vi "final_control_mk4_022525.vi"() -> ()   [LabVIEW 2023]
doc: "Simplified example program for initializing the COM port, determining the data frame of up to 26 Alicats, acquiring the data of the same number of Alicats, displaying the data of the one with the selected unit ID, and writing a setpoint to the same selected unit ID.\n\nThis is a slightly more feature rich version of the Alicat Simplified Driver Example, and contains an example of a method for interfacing with up to 26 Alicats on a single COM port by means of for loops with shift registers to handle sequential commands to each included Alicat. This also contains a method to write a setpoint to the same selected unit.\n\nIf coding for multiple Alicats on a single COM port without the use of for loops with shift registers, ensure that each Alicat command is executed sequentially. Alicat's RS-232/485 does not work if multiple devices are responding simultaneously."
uses:
  <vilib>/Platform/TimedLoop/XDataNode/timing_clust.ctl
  <vilib>/Platform/TimedLoop/XDataNode/nitl_modes.ctl
  <vilib>/Platform/TimedLoop/XDataNode/wakeup.ctl
  <vilib>/DAQmx/write.llb/DAQmx Write (Analog 1D DBL NChan 1Samp).vi
  <vilib>/DAQmx/read.llb/DAQmx Read (Analog 1D DBL 1Chan NSamp).vi
  <extravilib>/ChannelInstances/Tag-bool/Read With Abort.vi
  <extravilib>/ChannelInstances/Tag-bool/Write With Abort.vi
  <vilib>/Utility/file.llb/Write Delimited Spreadsheet (string).vi
  <extravilib>/ChannelInstances/Tag-bool/Instantiate.vi
  <vilib>/Utility/file.llb/Read Delimited Spreadsheet (DBL).vi
  <extravilib>/ChannelInstances/Tag-bool/EndpointRead.vi
  <vilib>/DAQmx/miscellaneous.llb/DAQmx Fill In Error Info.vi
  <extravilib>/ChannelInstances/Tag-bool/Endpoint.vi
  <vilib>/platform/TimedLoop/XDataNode/XDataNode.xnode
  <vilib>/Platform/TimedLoop/XDataNode/XDNodeRunTimeDep.lvlib
  <extravilib>/ChannelInstances/Tag-bool.lvlib
panel:
  in  "Tab Control":enum32{"Page 1", "Page 2"}(tab)
  in  "COM Port Settings":T1={"Baud Rate"=enum."19200", "VISA Sesssion In"="COM1"}
  out "Range Exceeded":bool
  out "Error Present":bool
  out "Error Text":string
  out "Elapsed Time [ms]\n(all units)":dbl caption="Elapsed Time (s)"
  in  "Minimum time between \nreadings [ms] (all units)":u32
  in  "Device ID's \nto Include:":T2={"A"=TRUE, "B"=FALSE, "C"=FALSE, "D"=FALSE, "E"=FALSE, "F"=FALSE, "G"=FALSE, "H"=FALSE, "I"=FALSE, "J"=FALSE, "K"=FALSE, "L"=FALSE, "M"=FALSE, "N"=FALSE, "O"=FALSE, "P"=FALSE, "Q"=FALSE, "R"=FALSE, "S"=FALSE, "T"=FALSE, "U"=FALSE, "V"=FALSE, "W"=FALSE, "X"=FALSE, "Y"=FALSE, "Z"=FALSE}
  out "Active Device":u16(ring) items=["A", "B", "C", "D", "E", "F"]
  out "Meas. Data (for active device)":T3
  in  "Write File":path=path "C:/Users/gtmiller/Downloads/Alicat LabVIEW 2014_2v1/Test.csv"
  in  "Hold Time [min]":dbl=17.0 min=17.0
  out "Global Start Time":i64
  out "N":i32
  out "Iteration Duration":i64
  in  "Read File":path
  in  "End Program":bool
  out "len_SP":i32
  out "Setpoints":dbl[][](array[numeric])=[[4.2, 3.3], [69.0, 4.2]]
  out "Z":dbl[](array[numeric])
  out "ASP":dbl
  out "BSP":dbl
  out "CSP":dbl
  out "DSP":dbl
  out "ESP":dbl
  out "FSP":dbl
  out "N_i_read":dbl
  out "N_read":i32
  out "read count":dbl=2.0
  out "Actual Start [i]":i64
  out "T_SCh":string[](array[string])
  out "Iter_Start_Time":string
  out "Iter_#":string
  out "V_D":string
  out "V_H":string
  # "Totalizer Timer"
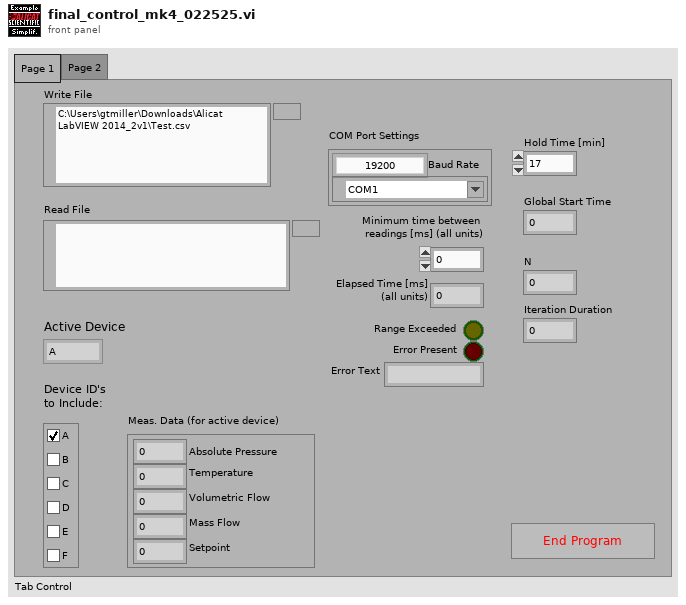
[diagram p1: front panel]
types:
  T1 = cluster{"Baud Rate":enum8{"2400", "9600", "19200", "38400", "57600", "115200", "Unknown"}, "VISA Sesssion In":refnum<visa-resource-name>}
  T2 = cluster{"A":bool, "B":bool, "C":bool, "D":bool, "E":bool, "F":bool, "G":bool, "H":bool, "I":bool, "J":bool, "K":bool, "L":bool, "M":bool, "N":bool, "O":bool, "P":bool, "Q":bool, "R":bool, "S":bool, "T":bool, "U":bool, "V":bool, "W":bool, "X":bool, "Y":bool, "Z":bool}
  T3 = cluster{"Absolute Pressure":dbl, "Gauge/Diff. Pressure":dbl, "Barometric Pressure":dbl, "Temperature":dbl, "Volumetric Flow":dbl, "Mass Flow":dbl, "Setpoint":dbl, "Valve Drive":dbl, "Totalizer":dbl, "[hr]":dbl, "[min]":dbl, "[sec]":dbl, "Totalizer Average Flow":dbl, "Totalizer Peak Flow":dbl, "Gas selected":string}
  T4 = cluster{"Unit ID":string, "Baud Rate":enum8{"2400", "9600", "19200", "38400", "57600", "115200", "Unknown"}, "VISA Sesssion In":refnum<visa-resource-name>}
  T5 = typedef "XDNodeRunTimeDep.lvlib/timing_clust.ctl" = cluster{"Expected End [f-1]":u64, "Actual End [f-1]":u64, "Finished Late? [f-1]":bool, "Expected End [i-1]":u64, "Actual End [i-1]":u64, "Finished Late? [i-1]":bool, "Expected Start [i]":u64, "Actual Start [i]":u64, "Expected Start [f]":u64, "Actual Start [f]":u64, "Source Name":string, "Structure Name":string, "Period":i64, "Deadline":i64, "Offset":i64, "Start":i64, "Priority":i32, "Timeout":i32, "Mode":T6, "Wakeup Reason":T7, "Error":errorcluster, "Source Type":string, "Secondary Source Type":string, "Global End Time":u64, "Global Start Time":u64, "Frame Duration":u64, "Iteration Duration":u64, "Assigned CPU":i32, "I/O Scan Engine Mode":u32}
  T6 = typedef "XDNodeRunTimeDep.lvlib/nitl_modes.ctl" = enum32{"No Change", "Process missed periods, maintain original phase", "Discard missed periods, maintain original phase", "Process missed periods, ignore original phase", "Discard missed periods, ignore original phase"}
  T7 = typedef "XDNodeRunTimeDep.lvlib/wakeup.ctl" = enum32{"Normal", "Aborted", "Asynchronous wakeup", "Timing source error", "Timed loop error", "Timeout"}
  T8 = enum8{"2400", "9600", "19200", "38400", "57600", "115200", "Unknown"}
  T9 = cluster{"Absolute Pressure":bool, "Gauge/Diff. Pressure":bool, "Barometric Pressure":bool, "Temperature":bool, "Volumetric":bool, "Mass":bool, "Setpoint":bool, "Valve Drive":bool, "Totalizer":bool, "Totalizer Timer":bool, "Totalizer Average Flow":bool, "Totalizer Peak Flow":bool, "Gas Selected":bool, "Tot. Timer Format":u16}
  T10 = cluster{"Controller Full Scale":dbl, "Controller Select":u16, "Control Range":enum16{"Normal", "Inverted", "Bidirectional", "Unknown"}}
  T11 = typedef "Tag-bool.lvlib/))Channel.ctl" = refnum<queue>
  T12 = cluster{"Controller Full Scale":dbl, "Controller Select":u16, "Control Range":enum16{"Normal", "Inverted", "Bidirectional", "Unknown"}}[]
diagram:
  n1 = for {
    N: 1 -> [_]
    # "Initialize Data Hold Array"
    # "All successive for loops to perform\nthe same task to all devices on the\nCOM port can make use of the for\nloop's auto-indexing feature"
    # "Set to run 26 times\n(once per letter)"
    # "Acquisition of data from multiple Alicats on a single serial line requires that the commands and returns are performed sequentially.\nThis is performed using for loops to gather and index the data in a sequential manner, but it can also be done with duplicated VI's called\nsequentially (but this becomes much more tedious if talking to more than 2 devices on a given COM port)."
    # "Numbers paired with Unit ID's included begin at\n0 for ease of use later on with for loop indexes"
    # "Get array of unit ID's and populate the Unit ID control before next step"
    # "Needs to be set before running software ->"
    # "Close the VISA session"
    # "Initialize the Com port\n(cluster bundle/unbundle\nused to provide Sub-VI \nwith the expected input)"
    n2 = Unbundle("COM Port Settings") -> ("Baud Rate"=w34:T8, "VISA Sesssion In"=w33:refnum<visa-resource-name>)
    n3 = Bundle(cluster=T4 {"Unit ID"="A", "Baud Rate"=enum."19200", "VISA Sesssion In"="COM1"} ("Communication Settings"), "Baud Rate"=w34, "VISA Sesssion In"=w33) -> (w32:T4)  [unwired: 1 in]
    n4 = Cluster To Array(cluster="Device ID's \nto Include:") -> (array=w28:bool[])
    n5 = call "COM Port Initialization.vi"("error in (no error)"=errorcluster {"status"=FALSE, "code"=0, "source"=""}, "Communication Settings"=w32) -> ("error out"=w25:errorcluster, "VISA Session Out"=w24:refnum<visa-resource-name>)  [unwired: 8 in]
    n6 = for {
      N: 6 -> [_]
      tunnel: "ABCDEF" -> [w516]
      tunnel: w28 -> [w509] mode=indexing
      shift-right: [w508] -> _
      shift-left: u16 0 ("length (rest)") -> [w514]
      shift-right: [w513] -> w22
      shift-left: cluster{string, u16}[] [] -> [w512]
      tunnel: w25 -> [w507]
      tunnel: w24 -> [w506]
      tunnel: [w507] -> w15
      tunnel: [w506] -> w23
      i -> [w515]
      # "Generate array of Device ID's, with sequential ID's"
      n7 = Equal?(x=w509, y=TRUE) -> (x = y?=w511:bool)
      n8 = case shown="True" w511 {
        tunnel: w516 -> [_ w527]
        tunnel: w515 -> [_ w526]
        tunnel: w514 -> [w517 w519]
        tunnel: [w518 w522] -> w513
        tunnel: w512 -> [w518 w520]
        tunnel: [w517 w523] -> w508
        frame False {
          # "ID was not included"
        }
        frame True {
          # "ID was included"
          n9 = String Subset(string=w527, offset (0)=w526, length (rest)=1 ("length (rest)")) -> (substring=w524:string)
          n10 = Bundle(w524, "length (rest)"=w519) -> (w521:cluster{string, "length (rest)":u16})  [unwired: 1 in]
          n11 = Increment(x=w519) -> (x+1=w523:u16)
          n12 = Build Array (concatenate)(w520, w521) -> (w522:cluster{string, "length (rest)":u16}[])
        }
      }
    }
    n13 = property on="Active Device" class="Ring (strict)"(error in=w15, "StringsAndValues[]"=w22) -> (error out=w14:errorcluster)  [unwired: 1 in, 1 out]
    n14 = for {
      tunnel: w23 -> [w504]
      tunnel: [w501] -> w19
      tunnel: w14 -> [w505]
      tunnel: [w500] -> w18
      tunnel: w22 -> [w502] mode=indexing
      tunnel: [w503] -> w21 mode=indexing
      tunnel: [w493] -> w20 mode=indexing
      tunnel: [w499] -> w17 mode=indexing
      tunnel: [nan ("Setpoint")] -> w16 mode=indexing
      tunnel: [w492] -> w13 mode=indexing
      # "Get measurement formats, unit ID's and the controller info"
      n15 = Unbundle(w502) -> (w493:string)  [unwired: 1 out]
      n16 = call "Read Measurement Format.vi"("Unit ID (A)"=w493, "error in"=w505, "VISA Session In"=w504) -> ("error out"=w496:errorcluster, "Data Frame Format"=w503:T9, "VISA Session Out"=w497:refnum<visa-resource-name>)  [unwired: 6 in]
      n17 = property on="Active Device" class="Ring (strict)" props=["Value"]() -> ()  [unwired: 2 in, 3 out]
      n18 = call "Read Software Version.vi"("Unit ID (A)"=w493, "error in"=w496, "VISA Session In"=w497) -> ("error out"=w495:errorcluster, "Software Version"=w492:u8, "VISA Session Out"=w494:refnum<visa-resource-name>)  [unwired: 6 in]
      n19 = call "Read Controller Info.vi"("Unit ID (A)"=w493, "error in"=w495, "Software Version"=w492, "VISA Session In"=w494) -> ("error out"=w500:errorcluster, "Controller Info out"=w499:T10, "VISA Session Out"=w501:refnum<visa-resource-name>)  [unwired: 4 in, 1 out]
    }
    n20 = Multiply(x="Hold Time [min]", y=60000.0) -> (x*y=w2:dbl)
    n21 = node-c288(w2) -> (w43:T5)  [unwired: 3 in]
    n22 = timed-loop "Write Data" {
      timing: w43 -> [_]
      timing-out: [_] -> w42
      tunnel: [w54] -> w9
      tunnel: "Write File" -> [w53]
      i -> [w66]
      stop <- w194 stop-if-true
      n23 = timed-sequence {
        timing: _ -> [_]
        timing-out: _ -> [_]
        tunnel: [w56] -> w54
        tunnel: w53 -> [w55]
        n24 = timed-flat-sequence {
          tunnel: [w189] -> w56
          tunnel: w55 -> [w190]
          frame #0 {
            w59 = u16 0 items=["A", "B", "C", "D", "E", "F"]
            n25 = node-c288() -> (→"Global Start Time":i64, →"Iteration Duration":i64)  [unwired: 1 in]
            n26 = local read "Setpoints"() -> (w68:dbl[][])
            n27 = Index Array(array=w68, index (row)=w66, index (col)=0 ("index (row)")) -> (element=w64:dbl)
            "ASP" <- w64
            n28 = local read "Z"() -> (w62:dbl[])
            n29 = Replace Array Subset(array=w62, new element #1=w64, index #1=0 ("index"), new element #2=w59, index #2=1 ("index")) -> (w63:dbl[])
            n30 = local write "Z"(w63) -> ()
            n31 = node-c288(i64 2000 ("Start")) -> ()  [unwired: 1 out]
            "N" <- w66
          }
          frame #1 {
            w77 = u16 1 items=["A", "B", "C", "D", "E", "F"]
            n32 = node-c288() -> ()  [unwired: 1 in, 1 out]
            n33 = local read "Setpoints"() -> (w85:dbl[][])
            n34 = local read "N"() -> (w78:i32)
            n35 = Index Array(array=w85, index (row)=w78, index (col)=1 ("index (row)")) -> (element=w82:dbl)
            "BSP" <- w82
            n36 = local read "Z"() -> (w80:dbl[])
            n37 = Replace Array Subset(array=w80, new element #1=w82, index #1=0 ("index"), new element #2=w77, index #2=1 ("index")) -> (w81:dbl[])
            n38 = call-poly <vilib>:"DAQmx Write.vi"("task/channels in"=refnum<k21> "Valve_cont", "data"=dbl[] [5.0, 5.0]) -> ()  [unwired: 11 in, 3 out]
            n39 = local write "Z"(w81) -> ()
            n40 = node-c288(i64 2000 ("Start")) -> ()  [unwired: 1 out]
          }
          frame #2 {
            w111 = u16 2 items=["A", "B", "C", "D", "E", "F"]
            n41 = node-c288() -> ()  [unwired: 1 in, 1 out]
            n42 = local read "Setpoints"() -> (w94:dbl[][])
            n43 = local read "N"() -> (w93:i32)
            n44 = Index Array(array=w94, index (row)=w93, index (col)=2 ("index (row)")) -> (element=w115:dbl)
            "CSP" <- w115
            n45 = Index Array(array=w94, index (row)=w93, index (col)=6 ("disabled index (col)")) -> (element=w92:dbl)
            n46 = Index Array(array=w94, index (row)=w93, index (col)=7 ("disabled index (col)")) -> (element=w91:dbl)
            n47 = local read "Z"() -> (w113:dbl[])
            n48 = Subtract(x=5.0, y=w92) -> (x-y=w108:dbl)
            n49 = Subtract(x=5.0, y=w91) -> (x-y=w103:dbl)
            n50 = Replace Array Subset(array=w113, new element #1=w115, index #1=0 ("index"), new element #2=w111, index #2=1 ("index")) -> (w114:dbl[])
            n51 = Multiply(x=w108, y=0.33) -> (x*y=w106:dbl)
            n52 = Multiply(x=w103, y=0.33) -> (x*y=w101:dbl)
            n53 = local write "Z"(w114) -> ()
            n54 = Subtract(x=5.0, y=w106) -> (x-y=w96:dbl)
            n55 = Subtract(x=5.0, y=w101) -> (x-y=w97:dbl)
            n56 = Build Array(w96, w97) -> (w95:dbl[])
            n57 = call-poly <vilib>:"DAQmx Write.vi"("task/channels in"=refnum<k21> "Valve_cont", "data"=w95) -> ()  [unwired: 11 in, 3 out]
            n58 = node-c288(i64 2000 ("Start")) -> ()  [unwired: 1 out]
          }
          frame #3 {
            w143 = u16 3 items=["A", "B", "C", "D", "E", "F"]
            n59 = node-c288() -> ()  [unwired: 1 in, 1 out]
            n60 = local read "Setpoints"() -> (w126:dbl[][])
            n61 = local read "N"() -> (w125:i32)
            n62 = Index Array(array=w126, index (row)=w125, index (col)=3 ("index (row)")) -> (element=w147:dbl)
            "DSP" <- w147
            n63 = Index Array(array=w126, index (row)=w125, index (col)=6 ("disabled index (col)")) -> (element=w124:dbl)
            n64 = Index Array(array=w126, index (row)=w125, index (col)=7 ("disabled index (col)")) -> (element=w123:dbl)
            n65 = local read "Z"() -> (w145:dbl[])
            n66 = Subtract(x=5.0, y=w124) -> (x-y=w140:dbl)
            n67 = Subtract(x=5.0, y=w123) -> (x-y=w135:dbl)
            n68 = Replace Array Subset(array=w145, new element #1=w147, index #1=0 ("index"), new element #2=w143, index #2=1 ("index")) -> (w146:dbl[])
            n69 = Multiply(x=w140, y=0.67) -> (x*y=w138:dbl)
            n70 = Multiply(x=w135, y=0.67) -> (x*y=w133:dbl)
            n71 = local write "Z"(w146) -> ()
            n72 = Subtract(x=5.0, y=w138) -> (x-y=w128:dbl)
            n73 = Subtract(x=5.0, y=w133) -> (x-y=w129:dbl)
            n74 = Build Array(w128, w129) -> (w127:dbl[])
            n75 = call-poly <vilib>:"DAQmx Write.vi"("task/channels in"=refnum<k21> "Valve_cont", "data"=w127) -> ()  [unwired: 11 in, 3 out]
            n76 = node-c288(i64 2000 ("Start")) -> ()  [unwired: 1 out]
          }
          frame #4 {
            w164 = u16 4 items=["A", "B", "C", "D", "E", "F"]
            n77 = node-c288() -> ()  [unwired: 1 in, 1 out]
            n78 = local read "Setpoints"() -> (w158:dbl[][])
            n79 = local read "N"() -> (w157:i32)
            n80 = Index Array(array=w158, index (row)=w157, index (col)=4 ("index (row)")) -> (element=w168:dbl)
            "ESP" <- w168
            n81 = Index Array(array=w158, index (row)=w157, index (col)=6 ("disabled index (col)")) -> (element=w160:dbl)
            n82 = Index Array(array=w158, index (row)=w157, index (col)=7 ("disabled index (col)")) -> (element=w159:dbl)
            n83 = local read "Z"() -> (w166:dbl[])
            n84 = Build Array(w160, w159) -> (w156:dbl[])
            n85 = Replace Array Subset(array=w166, new element #1=w168, index #1=0 ("index"), new element #2=w164, index #2=1 ("index")) -> (w167:dbl[])
            n86 = call-poly <vilib>:"DAQmx Write.vi"("task/channels in"=refnum<k21> "Valve_cont", "data"=w156) -> ()  [unwired: 11 in, 3 out]
            n87 = local write "Z"(w167) -> ()
            n88 = node-c288(i64 2000 ("Start")) -> ()  [unwired: 1 out]
          }
          frame #5 {
            w178 = u16 5 items=["A", "B", "C", "D", "E", "F"]
            n89 = node-c288() -> ()  [unwired: 1 in, 1 out]
            n90 = local read "N"() -> (w176:i32)
            n91 = local read "Setpoints"() -> (w181:dbl[][])
            n92 = local read "Z"() -> (w180:dbl[])
            n93 = Index Array(array=w181, index (row)=w176, index (col)=5 ("index (row)")) -> (element=w177:dbl)
            "FSP" <- w177
            n94 = Replace Array Subset(array=w180, new element #1=w177, index #1=0 ("index"), new element #2=w178, index #2=1 ("index")) -> (w179:dbl[])
            n95 = local write "Z"(w179) -> ()
            n96 = node-c288(i64 2000 ("Start")) -> ()  [unwired: 1 out]
          }
          frame #6 {
            n97 = node-c288() -> ()  [unwired: 1 in, 1 out]
            n98 = local read "len_SP"() -> (w193:i32)
            n99 = Subtract(x=w193, y=1) -> (x-y=w196:i32)
            n100 = local read "N"() -> (w192:i32)
            n101 = Equal?(x=w192, y=w196) -> (x = y?=w195:bool)
            n102 = Or(x="End Program", y=w195) -> (x .or. y?=w194:bool)
            n103 = call <extravilib>:"Write.vi"("element"=w194) -> ("channel"=w189:T11)  [unwired: 1 out]
            n104 = while {
              tunnel: w190 -> [w212]
              tunnel: w189 -> [w206]
              i -> [w202]
              stop <- w201 stop-if-true
              w207 = 42.0 ("y")
              # "Read Data"
              n105 = local read "N_i_read"() -> (w199:dbl)
              n106 = node-c288(w199) -> (w214:T5)  [unwired: 3 in]
              n107 = timed-loop {
                timing: w214 -> [_]
                timing-out: [_] -> w213
                tunnel: w212 -> [w216]
                tunnel: w206 -> [w215]
                i -> [w243]
                stop <- w443 stop-if-true
                n108 = timed-sequence {
                  timing: _ -> [_]
                  timing-out: _ -> [_]
                  tunnel: w216 -> [w223]
                  tunnel: w215 -> [w217]
                  n109 = timed-flat-sequence {
                    tunnel: w223 -> [w246]
                    tunnel: [w246] -> w222
                    tunnel: w222 -> [w286]
                    tunnel: [w286] -> w221
                    tunnel: w221 -> [w325]
                    tunnel: [w325] -> w220
                    tunnel: w220 -> [w364]
                    tunnel: [w364] -> w219
                    tunnel: w219 -> [w403]
                    tunnel: [w403] -> w218
                    tunnel: w218 -> [w450]
                    tunnel: w217 -> [w449]
                    frame #0 {
                      w235 = i16 2 ("precision (6)")
                      w242 = u16 5 items=["A", "B", "C", "D", "E", "F"]
                      w250 = u16 0 items=["A", "B", "C", "D", "E", "F"]
                      w251 = i16 6 ("precision (6)")
                      n110 = node-c288() -> (→"Actual Start [i]":i64)  [unwired: 1 in]
                      n111 = local read "Setpoints"() -> (w232:dbl[][])
                      n112 = local read "Setpoints"() -> (w226:dbl[][])
                      n113 = local read "Meas. Data (for active device)"() -> (w258:T3)
                      n114 = call-poly <vilib>:"DAQmx Read.vi"("task/channels in"=refnum<k21> "T_SCh") -> ("data"=w240:dbl[])  [unwired: 12 in, 2 out]
                      n115 = local read "Actual Start [i]"() -> (w236:i64)
                      n116 = local read "N"() -> (w227:i32)
                      n117 = Index Array(array=w232, index (row)=w227, index (col)=6 ("disabled index (col)")) -> (element=w231:dbl)
                      n118 = Index Array(array=w226, index (row)=w227, index (col)=7 ("disabled index (col)")) -> (element=w228:dbl)
                      n119 = local read "ASP"() -> (w244:dbl)
                      n120 = Unbundle(w258) -> ("Absolute Pressure"=w271:dbl, "Temperature"=w267:dbl, "Volumetric Flow"=w257:dbl, "Mass Flow"=w268:dbl, "Setpoint"=w269:dbl)  [unwired: 10 out]
                      n121 = local read "Z"() -> (w254:dbl[])
                      n122 = Number To Fractional String(number=w271, precision (6)=w251) -> (F-format string=w266:string)  [unwired: 2 in]
                      n123 = Number To Fractional String(number=w267, precision (6)=w251) -> (F-format string=w265:string)  [unwired: 2 in]
                      n124 = Number To Fractional String(number=w257, precision (6)=w251) -> (F-format string=w264:string)  [unwired: 2 in]
                      n125 = Number To Fractional String(number=w268, precision (6)=w251) -> (F-format string=w263:string)  [unwired: 2 in]
                      n126 = Number To Fractional String(number=w269, precision (6)=w251) -> (F-format string=w262:string)  [unwired: 2 in]
                      n127 = Number To Fractional String(number=w240, precision (6)=w235) -> (F-format string=w238:string[])  [unwired: 2 in]
                      "T_SCh" <- w238
                      n128 = Number To Fractional String(number=w236, precision (6)=w235) -> (F-format string=w237:string)  [unwired: 2 in]
                      "Iter_Start_Time" <- w237
                      n129 = Number To Fractional String(number=w227, precision (6)=i16 0) -> (F-format string=w234:string)  [unwired: 2 in]
                      "Iter_#" <- w234
                      n130 = Number To Fractional String(number=w231) -> (F-format string=w230:string)  [unwired: 3 in]
                      "V_D" <- w230
                      n131 = Number To Fractional String(number=w228) -> (F-format string=w229:string)  [unwired: 3 in]
                      "V_H" <- w229
                      n132 = Replace Array Subset(array=w254, new element #1=w250, index #1=1 ("index"), new element #2=w244, index #2=0 ("index")) -> (w252:dbl[])
                      n133 = Number To Fractional String(number=w242, precision (6)=w251) -> (F-format string=w270:string)  [unwired: 2 in]
                      n134 = Get Date/Time In Seconds() -> (seconds since 1Jan1904=w256:timestamp)
                      n135 = Get Date/Time String(seconds (now)=w256, want seconds? (F)=TRUE) -> (date string=w255:string, time string=w272:string)  [unwired: 1 in]
                      n136 = local write "Z"(w252) -> ()
                      n137 = Build Array (concatenate)(w255, w272, w270, w266, w265, w264, w263, w262, w238, w237, w234, w230, w229) -> (w259:string[])
                      n138 = node-c288(i64 1000 ("Start")) -> ()  [unwired: 1 out]
                      n139 = call-poly <vilib>:"Write Delimited Spreadsheet.vi"("file path (dialog if empty)"=w246, "format (%s)"="%.6f" ("format (%.3f)"), "1D data"=w259, "append to file? (new file:F)"=TRUE, "delimiter (\\t)"="," ("delimiter (\\t)")) -> ()  [unwired: 9 in, 2 out]
                      "N_read" <- w243
                    }
                    frame #1 {
                      w283 = u16 0 items=["A", "B", "C", "D", "E", "F"]
                      w293 = u16 1 items=["A", "B", "C", "D", "E", "F"]
                      w294 = i16 6 ("precision (6)")
                      n140 = node-c288() -> ()  [unwired: 1 in, 1 out]
                      n141 = local read "Meas. Data (for active device)"() -> (w291:T3)
                      n142 = Unbundle(w291) -> ("Absolute Pressure"=w311:dbl, "Temperature"=w307:dbl, "Volumetric Flow"=w298:dbl, "Mass Flow"=w308:dbl, "Setpoint"=w309:dbl)  [unwired: 10 out]
                      n143 = Number To Fractional String(number=w311, precision (6)=w294) -> (F-format string=w306:string)  [unwired: 2 in]
                      n144 = Number To Fractional String(number=w307, precision (6)=w294) -> (F-format string=w305:string)  [unwired: 2 in]
                      n145 = Number To Fractional String(number=w298, precision (6)=w294) -> (F-format string=w304:string)  [unwired: 2 in]
                      n146 = Number To Fractional String(number=w308, precision (6)=w294) -> (F-format string=w303:string)  [unwired: 2 in]
                      n147 = Number To Fractional String(number=w309, precision (6)=w294) -> (F-format string=w302:string)  [unwired: 2 in]
                      n148 = local read "BSP"() -> (w284:dbl)
                      n149 = local read "T_SCh"() -> (w282:string[])
                      n150 = local read "Iter_Start_Time"() -> (w281:string)
                      n151 = local read "Iter_#"() -> (w280:string)
                      n152 = local read "V_D"() -> (w279:string)
                      n153 = local read "V_H"() -> (w278:string)
                      n154 = local read "Z"() -> (w290:dbl[])
                      n155 = Replace Array Subset(array=w290, new element #1=w293, index #1=1 ("index"), new element #2=w284, index #2=0 ("index")) -> (w289:dbl[])
                      n156 = Number To Fractional String(number=w283, precision (6)=w294) -> (F-format string=w310:string)  [unwired: 2 in]
                      n157 = Get Date/Time In Seconds() -> (seconds since 1Jan1904=w297:timestamp)
                      n158 = Get Date/Time String(seconds (now)=w297, want seconds? (F)=TRUE) -> (date string=w296:string, time string=w312:string)  [unwired: 1 in]
                      n159 = local write "Z"(w289) -> ()
                      n160 = Build Array (concatenate)(w296, w312, w310, w306, w305, w304, w303, w302, w282, w281, w280, w279, w278) -> (w299:string[])
                      n161 = node-c288(i64 1000 ("Start")) -> ()  [unwired: 1 out]
                      n162 = call-poly <vilib>:"Write Delimited Spreadsheet.vi"("file path (dialog if empty)"=w286, "format (%s)"="%.6f" ("format (%.3f)"), "1D data"=w299, "append to file? (new file:F)"=TRUE, "delimiter (\\t)"="," ("delimiter (\\t)")) -> ()  [unwired: 9 in, 2 out]
                    }
                    frame #2 {
                      w322 = u16 1 items=["A", "B", "C", "D", "E", "F"]
                      w332 = u16 2 items=["A", "B", "C", "D", "E", "F"]
                      w333 = i16 6 ("precision (6)")
                      n163 = node-c288() -> ()  [unwired: 1 in, 1 out]
                      n164 = local read "Meas. Data (for active device)"() -> (w328:T3)
                      n165 = Unbundle(w328) -> ("Absolute Pressure"=w350:dbl, "Temperature"=w346:dbl, "Volumetric Flow"=w337:dbl, "Mass Flow"=w347:dbl, "Setpoint"=w348:dbl)  [unwired: 10 out]
                      n166 = local read "CSP"() -> (w323:dbl)
                      n167 = Number To Fractional String(number=w350, precision (6)=w333) -> (F-format string=w345:string)  [unwired: 2 in]
                      n168 = Number To Fractional String(number=w346, precision (6)=w333) -> (F-format string=w344:string)  [unwired: 2 in]
                      n169 = Number To Fractional String(number=w337, precision (6)=w333) -> (F-format string=w343:string)  [unwired: 2 in]
                      n170 = Number To Fractional String(number=w347, precision (6)=w333) -> (F-format string=w342:string)  [unwired: 2 in]
                      n171 = Number To Fractional String(number=w348, precision (6)=w333) -> (F-format string=w341:string)  [unwired: 2 in]
                      n172 = local read "Z"() -> (w330:dbl[])
                      n173 = local read "T_SCh"() -> (w321:string[])
                      n174 = local read "Iter_Start_Time"() -> (w320:string)
                      n175 = local read "Iter_#"() -> (w319:string)
                      n176 = local read "V_D"() -> (w318:string)
                      n177 = local read "V_H"() -> (w317:string)
                      n178 = Replace Array Subset(array=w330, new element #1=w332, index #1=1 ("index"), new element #2=w323, index #2=0 ("index")) -> (w329:dbl[])
                      n179 = Number To Fractional String(number=w322, precision (6)=w333) -> (F-format string=w349:string)  [unwired: 2 in]
                      n180 = local write "Z"(w329) -> ()
                      n181 = Get Date/Time In Seconds() -> (seconds since 1Jan1904=w336:timestamp)
                      n182 = Get Date/Time String(seconds (now)=w336, want seconds? (F)=TRUE) -> (date string=w335:string, time string=w351:string)  [unwired: 1 in]
                      n183 = Build Array (concatenate)(w335, w351, w349, w345, w344, w343, w342, w341, w321, w320, w319, w318, w317) -> (w338:string[])
                      n184 = node-c288(i64 1000 ("Start")) -> ()  [unwired: 1 out]
                      n185 = call-poly <vilib>:"Write Delimited Spreadsheet.vi"("file path (dialog if empty)"=w325, "format (%s)"="%.6f" ("format (%.3f)"), "1D data"=w338, "append to file? (new file:F)"=TRUE, "delimiter (\\t)"="," ("delimiter (\\t)")) -> ()  [unwired: 9 in, 2 out]
                    }
                    frame #3 {
                      w361 = u16 2 items=["A", "B", "C", "D", "E", "F"]
                      w371 = u16 3 items=["A", "B", "C", "D", "E", "F"]
                      w372 = i16 6 ("precision (6)")
                      n186 = node-c288() -> ()  [unwired: 1 in, 1 out]
                      n187 = local read "Meas. Data (for active device)"() -> (w369:T3)
                      n188 = Unbundle(w369) -> ("Absolute Pressure"=w389:dbl, "Temperature"=w385:dbl, "Volumetric Flow"=w376:dbl, "Mass Flow"=w386:dbl, "Setpoint"=w387:dbl)  [unwired: 10 out]
                      n189 = local read "DSP"() -> (w362:dbl)
                      n190 = Number To Fractional String(number=w389, precision (6)=w372) -> (F-format string=w384:string)  [unwired: 2 in]
                      n191 = Number To Fractional String(number=w385, precision (6)=w372) -> (F-format string=w383:string)  [unwired: 2 in]
                      n192 = Number To Fractional String(number=w376, precision (6)=w372) -> (F-format string=w382:string)  [unwired: 2 in]
                      n193 = Number To Fractional String(number=w386, precision (6)=w372) -> (F-format string=w381:string)  [unwired: 2 in]
                      n194 = Number To Fractional String(number=w387, precision (6)=w372) -> (F-format string=w380:string)  [unwired: 2 in]
                      n195 = local read "T_SCh"() -> (w360:string[])
                      n196 = local read "Iter_Start_Time"() -> (w359:string)
                      n197 = local read "Iter_#"() -> (w358:string)
                      n198 = local read "V_D"() -> (w357:string)
                      n199 = local read "V_H"() -> (w356:string)
                      n200 = local read "Z"() -> (w368:dbl[])
                      n201 = Replace Array Subset(array=w368, new element #1=w371, index #1=1 ("index"), new element #2=w362, index #2=0 ("index")) -> (w367:dbl[])
                      n202 = Number To Fractional String(number=w361, precision (6)=w372) -> (F-format string=w388:string)  [unwired: 2 in]
                      n203 = Get Date/Time In Seconds() -> (seconds since 1Jan1904=w375:timestamp)
                      n204 = Get Date/Time String(seconds (now)=w375, want seconds? (F)=TRUE) -> (date string=w374:string, time string=w390:string)  [unwired: 1 in]
                      n205 = local write "Z"(w367) -> ()
                      n206 = Build Array (concatenate)(w374, w390, w388, w384, w383, w382, w381, w380, w360, w359, w358, w357, w356) -> (w377:string[])
                      n207 = node-c288(i64 1000 ("Start")) -> ()  [unwired: 1 out]
                      n208 = call-poly <vilib>:"Write Delimited Spreadsheet.vi"("file path (dialog if empty)"=w364, "format (%s)"="%.6f" ("format (%.3f)"), "1D data"=w377, "append to file? (new file:F)"=TRUE, "delimiter (\\t)"="," ("delimiter (\\t)")) -> ()  [unwired: 9 in, 2 out]
                    }
                    frame #4 {
                      w400 = u16 3 items=["A", "B", "C", "D", "E", "F"]
                      w410 = u16 4 items=["A", "B", "C", "D", "E", "F"]
                      w411 = i16 6 ("precision (6)")
                      n209 = node-c288() -> ()  [unwired: 1 in, 1 out]
                      n210 = local read "Meas. Data (for active device)"() -> (w408:T3)
                      n211 = Unbundle(w408) -> ("Absolute Pressure"=w428:dbl, "Temperature"=w424:dbl, "Volumetric Flow"=w415:dbl, "Mass Flow"=w425:dbl, "Setpoint"=w426:dbl)  [unwired: 10 out]
                      n212 = local read "ESP"() -> (w401:dbl)
                      n213 = Number To Fractional String(number=w428, precision (6)=w411) -> (F-format string=w423:string)  [unwired: 2 in]
                      n214 = Number To Fractional String(number=w424, precision (6)=w411) -> (F-format string=w422:string)  [unwired: 2 in]
                      n215 = Number To Fractional String(number=w415, precision (6)=w411) -> (F-format string=w421:string)  [unwired: 2 in]
                      n216 = Number To Fractional String(number=w425, precision (6)=w411) -> (F-format string=w420:string)  [unwired: 2 in]
                      n217 = Number To Fractional String(number=w426, precision (6)=w411) -> (F-format string=w419:string)  [unwired: 2 in]
                      n218 = local read "Iter_Start_Time"() -> (w398:string)
                      n219 = local read "Iter_#"() -> (w397:string)
                      n220 = local read "V_D"() -> (w396:string)
                      n221 = local read "V_H"() -> (w395:string)
                      n222 = local read "T_SCh"() -> (w399:string[])
                      n223 = local read "Z"() -> (w407:dbl[])
                      n224 = Replace Array Subset(array=w407, new element #1=w410, index #1=1 ("index"), new element #2=w401, index #2=0 ("index")) -> (w406:dbl[])
                      n225 = Number To Fractional String(number=w400, precision (6)=w411) -> (F-format string=w427:string)  [unwired: 2 in]
                      n226 = Get Date/Time In Seconds() -> (seconds since 1Jan1904=w414:timestamp)
                      n227 = Get Date/Time String(seconds (now)=w414, want seconds? (F)=TRUE) -> (date string=w413:string, time string=w429:string)  [unwired: 1 in]
                      n228 = local write "Z"(w406) -> ()
                      n229 = Build Array (concatenate)(w413, w429, w427, w423, w422, w421, w420, w419, w399, w398, w397, w396, w395) -> (w416:string[])
                      n230 = node-c288(i64 1000 ("Start")) -> ()  [unwired: 1 out]
                      n231 = call-poly <vilib>:"Write Delimited Spreadsheet.vi"("file path (dialog if empty)"=w403, "format (%s)"="%.6f" ("format (%.3f)"), "1D data"=w416, "append to file? (new file:F)"=TRUE, "delimiter (\\t)"="," ("delimiter (\\t)")) -> ()  [unwired: 9 in, 2 out]
                    }
                    frame #5 {
                      w439 = u16 4 items=["A", "B", "C", "D", "E", "F"]
                      w456 = u16 5 items=["A", "B", "C", "D", "E", "F"]
                      w457 = i16 6 ("precision (6)")
                      n232 = node-c288() -> ()  [unwired: 1 in, 1 out]
                      n233 = local read "Meas. Data (for active device)"() -> (w454:T3)
                      n234 = Unbundle(w454) -> ("Absolute Pressure"=w474:dbl, "Temperature"=w470:dbl, "Volumetric Flow"=w461:dbl, "Mass Flow"=w471:dbl, "Setpoint"=w472:dbl)  [unwired: 10 out]
                      n235 = local read "FSP"() -> (w447:dbl)
                      n236 = Number To Fractional String(number=w474, precision (6)=w457) -> (F-format string=w469:string)  [unwired: 2 in]
                      n237 = Number To Fractional String(number=w470, precision (6)=w457) -> (F-format string=w468:string)  [unwired: 2 in]
                      n238 = Number To Fractional String(number=w461, precision (6)=w457) -> (F-format string=w467:string)  [unwired: 2 in]
                      n239 = Number To Fractional String(number=w471, precision (6)=w457) -> (F-format string=w466:string)  [unwired: 2 in]
                      n240 = Number To Fractional String(number=w472, precision (6)=w457) -> (F-format string=w465:string)  [unwired: 2 in]
                      n241 = local read "Z"() -> (w453:dbl[])
                      n242 = local read "T_SCh"() -> (w438:string[])
                      n243 = local read "Iter_Start_Time"() -> (w437:string)
                      n244 = local read "Iter_#"() -> (w436:string)
                      n245 = local read "V_D"() -> (w435:string)
                      n246 = local read "V_H"() -> (w434:string)
                      n247 = Replace Array Subset(array=w453, new element #1=w456, index #1=1 ("index"), new element #2=w447, index #2=0 ("index")) -> (w452:dbl[])
                      n248 = local read "read count"() -> (w440:dbl)
                      n249 = Number To Fractional String(number=w439, precision (6)=w457) -> (F-format string=w473:string)  [unwired: 2 in]
                      n250 = local read "N_read"() -> (w444:i32)
                      n251 = Get Date/Time In Seconds() -> (seconds since 1Jan1904=w460:timestamp)
                      n252 = Get Date/Time String(seconds (now)=w460, want seconds? (F)=TRUE) -> (date string=w459:string, time string=w475:string)  [unwired: 1 in]
                      n253 = local write "Z"(w452) -> ()
                      n254 = Subtract(x=w440, y=1.0) -> (x-y=w442:dbl)
                      n255 = Build Array (concatenate)(w459, w475, w473, w469, w468, w467, w466, w465, w438, w437, w436, w435, w434) -> (w462:string[])
                      n256 = Equal?(x=w444, y=w442) -> (x = y?=w445:bool)
                      n257 = call-poly <vilib>:"Write Delimited Spreadsheet.vi"("file path (dialog if empty)"=w450, "format (%s)"="%.6f" ("format (%.3f)"), "1D data"=w462, "append to file? (new file:F)"=TRUE, "delimiter (\\t)"="," ("delimiter (\\t)")) -> ()  [unwired: 9 in, 2 out]
                      n258 = call <extravilib>:"Read.vi"("channel"=w449) -> ("element"=w446:bool)  [unwired: 1 in, 1 out]
                      n259 = Or(x=w445, y=w446) -> (x .or. y?=w443:bool)
                      n260 = node-c288() -> ()  [unwired: 1 in, 1 out]
                    }
                  }
                }
                n261 = node-c288() -> ()  [unwired: 1 in, 1 out]
                n262 = node-c288() -> ()  [unwired: 1 in, 1 out]
              }
              n263 = Equal?(x=w202, y=0.0) -> (x = y?=w204:bool)
              n264 = call <extravilib>:"Read.vi"("channel"=w206) -> ("element"=w203:bool)  [unwired: 1 in, 1 out]
              n265 = Or(x=w204, y=w203) -> (x .or. y?=w201:bool)
              n266 = node-c288(w213) -> ()  [unwired: 1 out]
              n267 = local read "Hold Time [min]"() -> (w210:dbl)
              n268 = Multiply(x=w210, y=60000.0) -> (x*y=w209:dbl)
              n269 = Subtract(x=w209, y=12000.0) -> (x-y=w200:dbl)
              n270 = Divide(x=w200, y=w207) -> (x/y=w198:dbl)
              "N_i_read" <- w198
              n271 = Wait (ms)(milliseconds to wait=w198) -> ()  [unwired: 1 out]
              "read count" <- w207
            }
            n272 = node-c288() -> ()  [unwired: 1 in, 1 out]
          }
        }
      }
      n273 = node-c288() -> ()  [unwired: 1 in, 1 out]
      n274 = node-c288() -> ()  [unwired: 1 in, 1 out]
    }
    n275 = while {
      shift-right: [w564] -> _
      shift-left: 0.0 ("Set Start Time (s)") -> [w567]
      shift-right: [w548] -> w37
      shift-left: w18 -> [w566]
      shift-right: [w549] -> w38
      shift-left: w19 -> [w565]
      tunnel: w20 -> [w541]
      shift-right: [w552] -> _
      shift-left: w21 -> [w559]
      shift-right: [w547] -> _
      shift-left: w17 -> [w545]
      shift-right: [w543] -> _
      shift-left: w16 -> [w542]
      shift-right: [w537] -> _
      shift-left: w13 -> [w537]
      tunnel: w9 -> [w535]
      stop <- w536 stop-if-true
      # "Set minimum time\nbetween loops"
      # "Acquire data for every device ID included at the requested data rate, then display only the selected device's data"
      n276 = call "Elapsed Time"("Set Start Time (s)"=w567) -> ("Get Start Time (s)"=w564:dbl, "Elapsed Time (s)"=w561:dbl)  [unwired: 11 in, 6 out]
      n277 = Wait (ms)(milliseconds to wait="Minimum time between \nreadings [ms] (all units)") -> ()  [unwired: 1 out]
      n278 = for {
        shift-right: [w596] -> w558
        shift-left: w566 -> [w599]
        shift-right: [w597] -> w557
        shift-left: w565 -> [w598]
        tunnel: w559 -> [w593] mode=indexing
        tunnel: w541 -> [w592] mode=indexing
        tunnel: [w591] -> w556 mode=indexing
        tunnel: [w590] -> w555 mode=indexing
        tunnel: [w589] -> w554 mode=indexing
        tunnel: [w588] -> w553 mode=indexing
        tunnel: [w587] -> w552 mode=indexing
        # "Acquire data for each device"
        n279 = call "Read Measurements.vi"("error in"=w599, "Data Frame Format In"=w593, "Unit ID (A)"=w592, "VISA Session In"=w598) -> ("error out"=w596:errorcluster, "Data Frame Format Out"=w587:T9, "Data Cluster"=w590:T3, "VISA Session Out"=w597:refnum<visa-resource-name>, "Unknown Dataframe Info"=w595:bool, "Error/Overrange/Unknown String"=w589:string, "Error Present"=w594:bool, "Range Exceeded"=w588:bool)
        n280 = Or(x=w595, y=w594) -> (x .or. y?=w591:bool)
      }
      n281 = Multiply(x=1000.0 ("y"), y=w561) -> (x*y=→"Elapsed Time [ms]\n(all units)":dbl)
      n282 = Reciprocal(x=w561) -> ()  [unwired: 1 out]
      n283 = local read "Z"() -> (w531:dbl[])
      n284 = Index Array(array=w531, index=1 ("index (row)")) -> (element=w529:dbl)
      "Active Device" <- w529
      n285 = To Long Integer(number=w529) -> (32bit integer=w539:i32)
      n286 = for {
        tunnel: w558 -> [w570]
        tunnel: [w569] -> w550
        tunnel: w557 -> [w571]
        tunnel: [w568] -> w551
        tunnel: w556 -> [w576] mode=indexing
        tunnel: w539 -> [w578]
        tunnel: w555 -> [w575] mode=indexing
        tunnel: w554 -> [w574] mode=indexing
        tunnel: w553 -> [w573] mode=indexing
        i -> [w577]
        # "Iterate over all sets of data, only display the one selected"
        n287 = Equal?(x=w578, y=w577) -> (x = y?=w572:bool)
        n288 = case shown="True" w572 {
          tunnel: w576 -> [_ w586]
          tunnel: w575 -> [_ w581]
          tunnel: w574 -> [_ w585]
          tunnel: w573 -> [_ w584]
          tunnel: w571 -> [w580 w582]
          tunnel: w570 -> [w579 w583]
          tunnel: [w579 w583] -> w569
          tunnel: [w580 w582] -> w568
          frame False {
            # "Do nothing"
          }
          frame True {
            # "Display data"
            "Range Exceeded" <- w584
            "Error Present" <- w586
            "Error Text" <- w585
            "Meas. Data (for active device)" <- w581
          }
        }
      }
      n289 = Index Array(array=w537, index=w539) -> (element=w538:u8)
      n290 = local read "Z"() -> (w534:dbl[])
      n291 = Index Array(array=w541, index=w539) -> (element=w540:string)
      n292 = Index Array(array=w545, index=w539) -> (element=w544:T10)
      n293 = Index Array(array=w542, index=w539) -> (element=w528:dbl)
      n294 = Index Array(array=w534, index=0) -> (element=w532:dbl)
      n295 = call "Write SetPoint_no prev.vi"("Setpoint"=w532, "Previous Setpoint"=w528, "Unit ID (A)"=w540, "error in"=w550, "Software Version"=w538, "Controller Info out"=w544, "VISA Session In"=w551) -> ("error out"=w548:errorcluster, "Controller Info out"=w546:T10, "VISA Session Out"=w549:refnum<visa-resource-name>)  [unwired: 1 in, 1 out]
      n296 = Replace Array Subset(array=w542, new element=w532, index=w539) -> (w543:dbl[])
      n297 = Replace Array Subset(array=w545, new element=w546, index=w539) -> (w547:T12)
      n298 = call <extravilib>:"Read.vi"("channel"=w535) -> ("element"=w536:bool)  [unwired: 1 in, 1 out]
    }
    n299 = call-poly <vilib>:"Write Delimited Spreadsheet.vi"("file path (dialog if empty)"="Write File", "1D data"=string[] ["Date", "Time [hh:mm:ss]", "Device ID", "Abs_P_MFC [psi]", "T_MFC [C]", "Volume Flow [LPM]", "Mass Flow [SLPM]", "SP_MFC [LPM]", "T_SCh", "Iter_Start_Time", "Iter_#", "V_D", "V_H"], "append to file? (new file:F)"=FALSE, "delimiter (\\t)"="," ("delimiter (\\t)")) -> ()  [unwired: 10 in, 2 out]
    n300 = VISA Close(VISA resource name=w38, error in (no error)=w37) -> (error out=w39:errorcluster)
    n301 = call <vilib>:"Simple Error Handler.vi"("error in (no error)"=w39) -> ()  [unwired: 4 in, 5 out]
    n302 = Initialize Array(0.0 ("element"), 2 ("dimension size")) -> (→"Z":dbl[])
    n303 = while "Hold Setpoints" {
      tunnel: w9 -> [w48]
      stop <- w49 stop-if-true
      n304 = call-poly <vilib>:"Read Delimited Spreadsheet.vi"("file path (dialog if empty)"="Read File", "start of read offset (chars.:0)"=1, "delimiter (\\t)"="," ("delimiter (\\t)")) -> ("all rows"=w46:dbl[][])  [unwired: 7 in, 5 out]
      "Setpoints" <- w46
      n305 = Array Size(array=w46) -> (size(s)=w51:i32[])
      n306 = call <extravilib>:"Read.vi"("channel"=w48) -> ("element"=w49:bool)  [unwired: 1 in, 1 out]
      n307 = Index Array(array=w51, index=0) -> (element=→"len_SP":i32)
    }
    n308 = node-c288(w42) -> ()  [unwired: 1 out]
  }
